vi "MenuConfig_LevelWrite.vi"(6 "Level.Label (\"\": Same as ID)":string, 8 "error in (no error)":errorcluster, 9 "Button.ID[]":string[](array[string]), 10 "Level.ID":string, 11 "MenuConfig":variant) -> (0 "error out":errorcluster, 3 "MenuConfig":variant)   [LabVIEW 2019, in "Menu Button.xctl"]
doc: "JSMA Module Template - Top Level UI 0.2.0.4\nRob Humfeld - Jet Engineering\nCopyright (c) 2019, Jet Engineering"
uses:
  Menu Button.xctl
  private/Level Config Cluster STYP.ctl
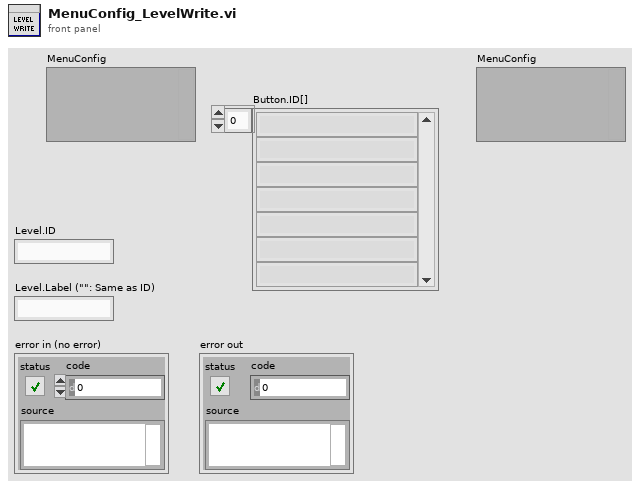
[diagram p1: front panel]
types:
  T1 = typedef "Menu Button.xctl/Level Config Cluster STYP.ctl" = cluster{"ID":string, "Label":string, "Button.ID[]":string[]}
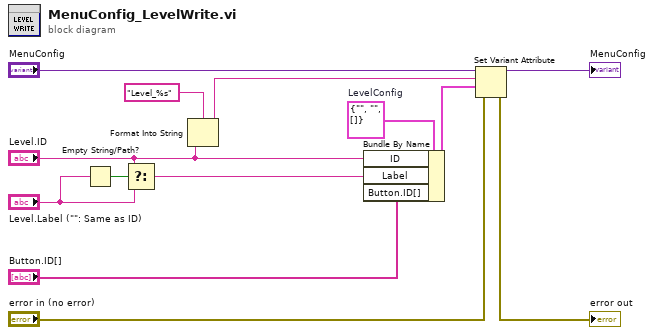
[diagram p0: block diagram]
diagram:
  w13 = T1 {"ID"="", "Label"="", "Button.ID[]"=[]}  # LevelConfig
  n1 = Empty String/Path?(string/path="Level.Label (\"\": Same as ID)") -> (empty?=w6:bool)
  n2 = Select(t="Level.ID", s=w6, f="Level.Label (\"\": Same as ID)") -> (s? t:f=w4:string)
  n3 = Format Into String(format string="Level_%s", "Level.ID") -> (resulting string=w1:string)  [unwired: 2 in, 1 out]
  n4 = Bundle By Name(cluster=w13, "ID"="Level.ID", "Label"=w4, "Button.ID[]"="Button.ID[]") -> (w11:T1)
  n5 = Set Variant Attribute(Variant="MenuConfig", name=w1, value=w11, error in="error in (no error)") -> (Variant out=→"MenuConfig":variant, error out=→"error out":errorcluster)  [unwired: 1 out]
